vi "ReversedEngineering RemoveThesePathes.vi"(1 "classesIn":path[](array[path]), 2 "removeThese":path[](array[path])) -> (15 "classesOut":path[](array[path]), 16 "Removed(Index-1*n)":i32[](array[numeric]))   [LabVIEW 2016]
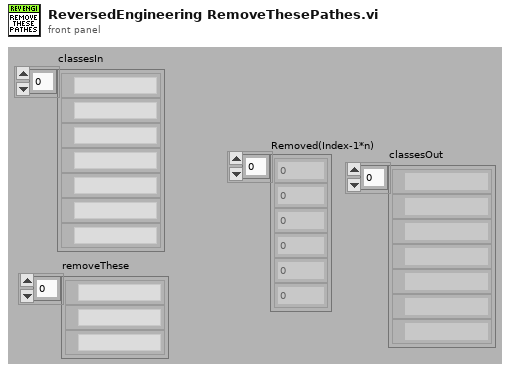
[diagram p1: front panel]
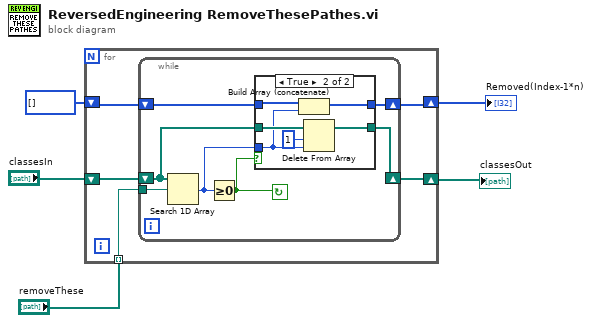
[diagram p0: block diagram]
diagram:
  n1 = for {
    tunnel: "removeThese" -> [w10] mode=indexing
    shift-right: [w8] -> w3
    shift-left: "classesIn" -> [w9]
    shift-right: [w7] -> w2
    shift-left: i32[] [] -> [w6]
    n2 = while {
      tunnel: w10 -> [w17]
      shift-right: [w14] -> w8
      shift-left: w9 -> [w15]
      shift-right: [w11] -> w7
      shift-left: w6 -> [w12]
      stop <- w16 continue-if-true
      n3 = Search 1D Array(1D array=w15, element=w17) -> (index of element=w13:i32)  [unwired: 1 out]
      n4 = Greater Or Equal To 0?(x=w13) -> (x >= 0?=w16:bool)
      n5 = case shown="True" w16 {
        tunnel: w15 -> [w19 w25]
        tunnel: w13 -> [_ w22]
        tunnel: [w19 w23] -> w14
        tunnel: w12 -> [w18 w20]
        tunnel: [w18 w21] -> w11
        frame False {
        }
        frame True {
          n6 = Build Array (concatenate)(w20, w22) -> (w21:i32[])
          n7 = Delete From Array(array=w25, length=1, index=w22) -> (array with subset deleted=w23:path[])  [unwired: 1 out]
        }
      }
    }
  }
  "classesOut" <- w3
  "Removed(Index-1*n)" <- w2
